vi "随机数文件作业.vi"() -> ()   [LabVIEW 2014]
uses:
  <vilib>/Utility/file.llb/Write To Spreadsheet File (DBL).vi
  <vilib>/Utility/file.llb/Read From Spreadsheet File (DBL).vi
panel:
  out "已排序的数组":dbl[](array[numeric])
  out "1D data 3":dbl[](array[numeric]) caption="正数" format="%0.2f"
  out "1D data 2":dbl[](array[numeric]) caption="负数" format="%0.2f"
  in  "停止创建原始数组":bool
  out "原始数组":dbl[](array[numeric])
  # "232142      梁植源      20141000335\n随机数文件，注释见程序框图"
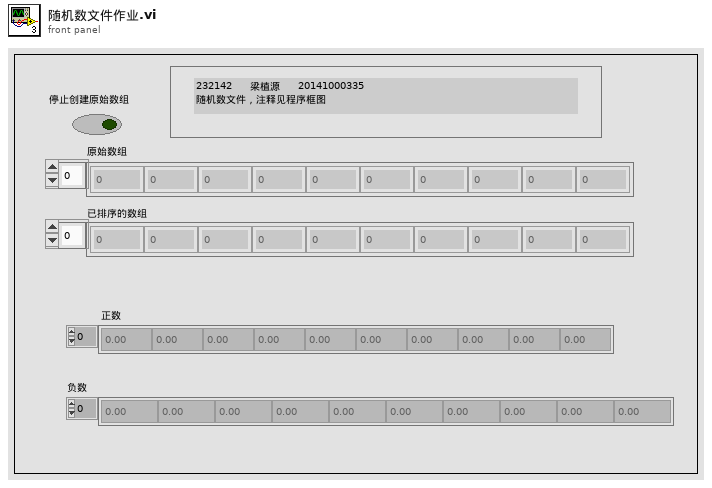
[diagram p1: front panel]
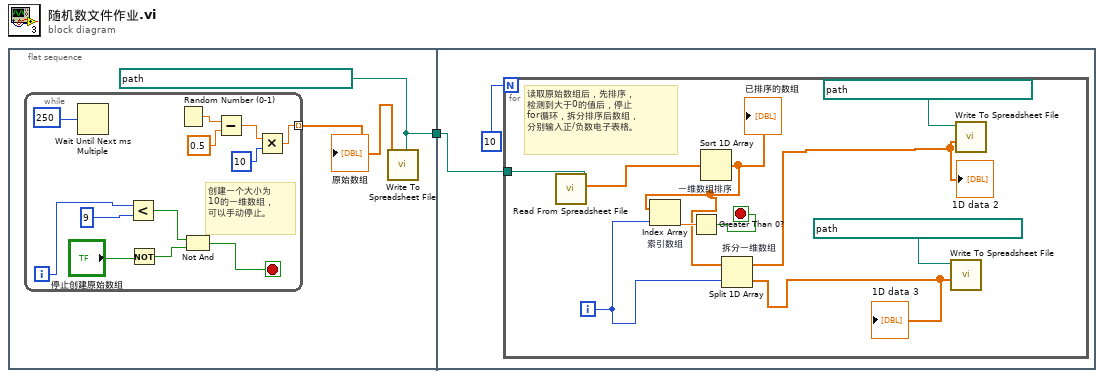
[diagram p0: block diagram]
diagram:
  n1 = flat-sequence {
    tunnel: [w3] -> w1
    tunnel: w1 -> [w16]
    frame #0 {
      w3 = path "C:/Users/wyman/Desktop/原始数据.xls"
      n2 = while {
        tunnel: [w4] -> w2 mode=indexing
        i -> [w10]
        stop <- w13 stop-if-true
        # "创建一个大小为\n10的一维数组，\n可以手动停止。"
        n3 = Wait Until Next ms Multiple(millisecond multiple=250) -> ()  [unwired: 1 out]
        n4 = Less?(x=w10, y=9) -> (x < y?=w12:bool)
        n5 = Not(x="停止创建原始数组") -> (.not. x?=w14:bool)
        n6 = Random Number (0-1)() -> (number: 0 to 1=w8:dbl)
        n7 = Not And(1:w14, 2:w12) -> (0:w13:bool)
        n8 = Subtract(x=w8, y=0.5) -> (x-y=w5:dbl)
        n9 = Multiply(x=w5, y=10) -> (x*y=w4:dbl)
      }
      "原始数组" <- w2
      n10 = call-poly <vilib>:"Write To Spreadsheet File.vi"("1D data"=w2, "file path (dialog if empty)"=w3) -> ()  [unwired: 6 in, 1 out]
    }
    frame #1 {
      n11 = for {
        N: 10 -> [_]
        tunnel: w16 -> [w27]
        i -> [w18]
        stop <- w23 stop-if-true
        # "读取原始数组后，先排序，\n检测到大于0的值后，停止\nfor循环，拆分排序后数组，\n分别输入正/负数电子表格。"
        n12 = call-poly <vilib>:"Read From Spreadsheet File.vi"("file path (dialog if empty)"=w27) -> ("first row"=w26:dbl[])  [unwired: 6 in, 4 out]
        n13 = Sort 1D Array "一维数组排序"(array=w26) -> (sorted array=w24:dbl[])
        "已排序的数组" <- w24
        n14 = Index Array "索引数组"(array=w24, index=w18) -> (element=w25:dbl)
        n15 = Greater Than 0?(x=w25) -> (x > 0?=w23:bool)
        n16 = Split 1D Array "拆分一维数组"(array=w24, index=w18) -> (first subarray=w21:dbl[], second subarray=w19:dbl[])
        "1D data 2" <- w21
        "1D data 3" <- w19
        n17 = call-poly <vilib>:"Write To Spreadsheet File.vi"("1D data"=w19, "file path (dialog if empty)"=path "C:/Users/wyman/Desktop/正数.xls") -> ()  [unwired: 6 in, 1 out]
        n18 = call-poly <vilib>:"Write To Spreadsheet File.vi"("1D data"=w21, "file path (dialog if empty)"=path "C:/Users/wyman/Desktop/负数.xls") -> ()  [unwired: 6 in, 1 out]
      }
    }
  }
